vi "Update Account Balance.vi"(8 "error in (no error)":errorcluster, 9 "Add or Subtract":enum16{"Add", "Subtract"}(ring)=enum."Subtract", 10 "Amount":string, 11 "PIN":string) -> (0 "error out":errorcluster, 2 "Message":string)   [LabVIEW 2025]
doc: "Updates Account Balance in the Accounts.csv file."
uses:
  <vilib>/Utility/file.llb/Read Delimited Spreadsheet (string).vi
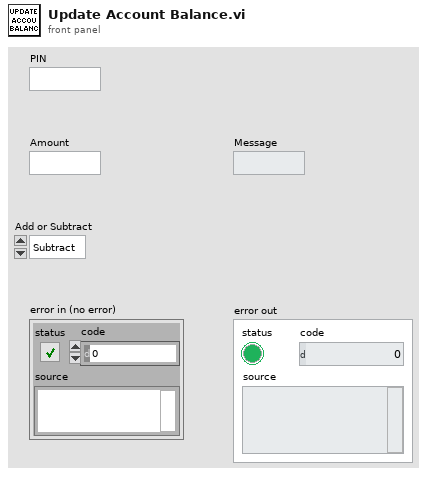
[diagram p1: front panel]
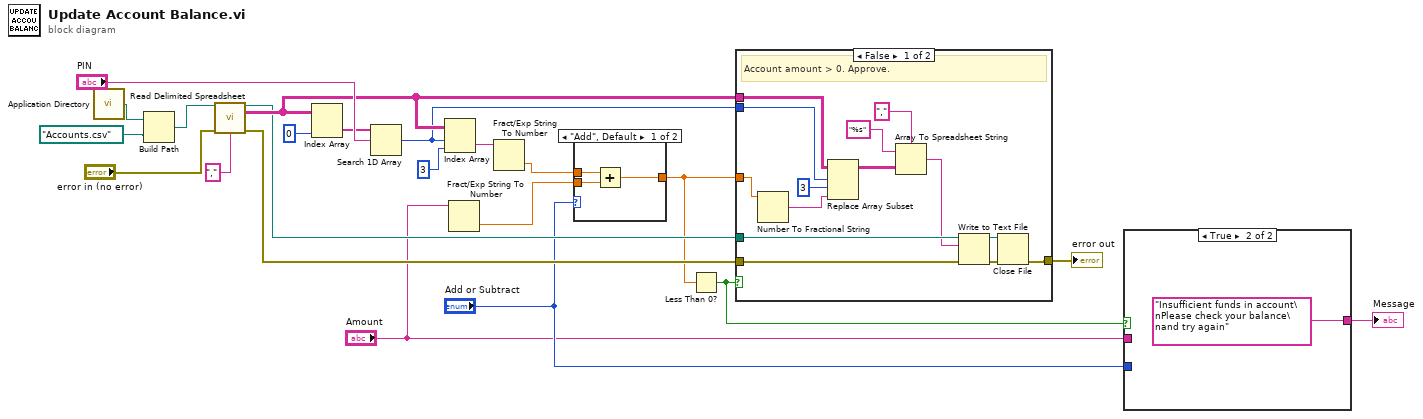
[diagram p0: block diagram]
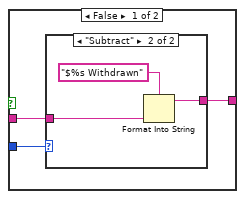
[diagram p2: hidden frame]
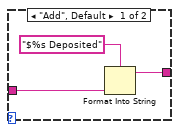
[diagram p3: hidden frame]
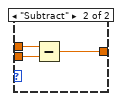
[diagram p4: hidden frame]
diagram:
  n1 = call <vilib>:"Application Directory.vi"() -> ("Application Directory"=w14:path)
  n2 = Build Path(base path=w14, name or relative path=path "Accounts.csv") -> (appended path=w12:path)
  n3 = call-poly <vilib>:"Read Delimited Spreadsheet.vi"("file path (dialog if empty)"=w12, "error in (no error)"="error in (no error)", "delimiter (\\t)"="," ("delimiter (\\t)")) -> ("new file path (Not A Path if cancelled)"=w8:path, "all rows"=w10:string[][], "error out"=w7:errorcluster)  [unwired: 7 in, 3 out]
  n4 = Index Array(array=w10, index (col)=0) -> (element=w13:string[])  [unwired: 1 in]
  n5 = Search 1D Array(1D array=w13, element="PIN") -> (index of element=w9:i32)  [unwired: 1 in]
  n6 = Index Array(array=w10, index (row)=w9, index (col)=3) -> (element=w20:string)
  n7 = Fract/Exp String To Number(string="Amount") -> (number=w21:dbl)  [unwired: 3 in, 1 out]
  n8 = Fract/Exp String To Number(string=w20) -> (number=w22:dbl)  [unwired: 3 in, 1 out]
  n9 = case shown="\"Add\", Default" "Add or Subtract" {
    tunnel: w22 -> [w25 w27]
    tunnel: w21 -> [w24 w26]
    tunnel: [w23 w28] -> w5
    frame "Add", Default {
      n10 = Add(x=w25, y=w24) -> (x+y=w23:dbl)
    }
    frame "Subtract" {
      n11 = Subtract(x=w27, y=w26) -> (x-y=w28:dbl)
    }
  }
  n12 = Less Than 0?(x=w5) -> (x < 0?=w4:bool)
  n13 = case shown="False" w4 {
    tunnel: w10 -> [w42 _]
    tunnel: w9 -> [w40 _]
    tunnel: w8 -> [w39 _]
    tunnel: w7 -> [w38 w43]
    tunnel: [w33 w43] -> w6
    tunnel: w5 -> [w31 _]
    frame False {
      # "Account amount > 0. Approve."
      n14 = Number To Fractional String(number=w31) -> (F-format string=w29:string)  [unwired: 3 in]
      n15 = Replace Array Subset(array=w42, new element=w29, index (row)=w40, index (col)=3 ("index")) -> (w37:string[][])
      n16 = Array To Spreadsheet String(delimiter (Tab)=",", array=w37, 3:"%s" ("format string")) -> (spreadsheet string=w30:string)
      n17 = Write to Text File(file (use dialog)=w39, text=w30, error in=w38) -> (refnum out=w34:refnum<file>, error out=w35:errorcluster)  [unwired: 1 in, 1 out]
      n18 = Close File(refnum=w34, error in=w35) -> (error out=w33:errorcluster)  [unwired: 1 out]
    }
    frame True {
      # "Account amount less than 0. Deny."
    }
  }
  "error out" <- w6
  n19 = case shown="True" w4 {
    tunnel: "Add or Subtract" -> [w46 _]
    tunnel: [w45 "Insufficient funds in account\nPlease check your balance\nand try again"] -> w2
    tunnel: "Amount" -> [w44 _]
    frame False {
      n20 = case shown="\"Subtract\"" w46 {
        tunnel: [w48 w51] -> w45
        tunnel: w44 -> [w47 w50]
        frame "Add", Default {
          n21 = Format Into String(format string="$%s Deposited", w47) -> (resulting string=w48:string)  [unwired: 2 in, 1 out]
        }
        frame "Subtract" {
          n22 = Format Into String(format string="$%s Withdrawn", w50) -> (resulting string=w51:string)  [unwired: 2 in, 1 out]
        }
      }
    }
    frame True {
    }
  }
  "Message" <- w2
